vi "Global stop.vi"() -> ()   [LabVIEW 2019]
panel:
  in  "Stop":bool
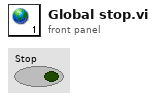
[diagram p1: front panel]
diagram:
